vi "BuildPlotsOneGraph.vi"(0 "PlotCommand":string, 1 "Desired Legends":string[](array[string]), 2 "Error Bar Type":T1=enum."Standard Error", 5 "Plotstyles":T3[](array[typedef]) {"LineType" min=1 max=6 step=1; "LineWidth" min=1 max=6 step=1; "PointSize" min=0 step=0.1}, 7 "PlotNamesNeed $$?":bool=TRUE, 9 "Plot Legends":string[](array[string]), 11 "PlotArray":cluster{dbl[], dbl[]}[](array[cluster]), 12 "Legend":string[](array[string]), 13 "Error Bar Cluster":T2[](array[typedef])) -> (4 "String out":string, 6 "Xspan":cluster{"Max":dbl, "Min":dbl}, 10 "Yspan":cluster{"Max":dbl, "Min":dbl})   [LabVIEW 2018]
uses:
  plotstyle.ctl
  Error_bars.ctl
  Error bar Type.ctl
  Results_plotter_Global.vi
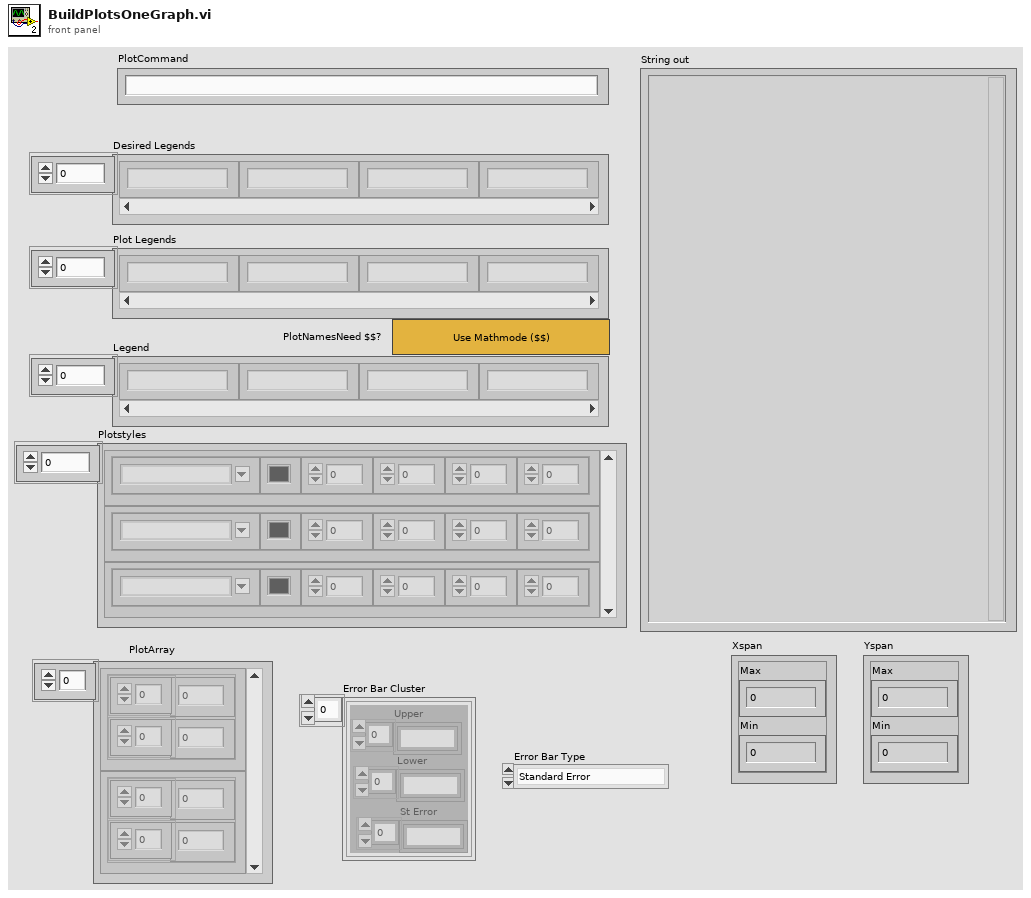
[diagram p1: front panel]
types:
  T1 = typedef "Error bar Type.ctl" = enum16{"None", "Standard Error", "Separate upper and lower"}
  T2 = typedef "Error_bars.ctl" = cluster{"Upper":string[], "Lower":string[], "St Error":string[]}
  T3 = typedef "plotstyle.ctl" = cluster{"Style":string, "Color":u32, "PointType":i32, "PointSize":sgl, "LineWidth":sgl, "LineType":u8}
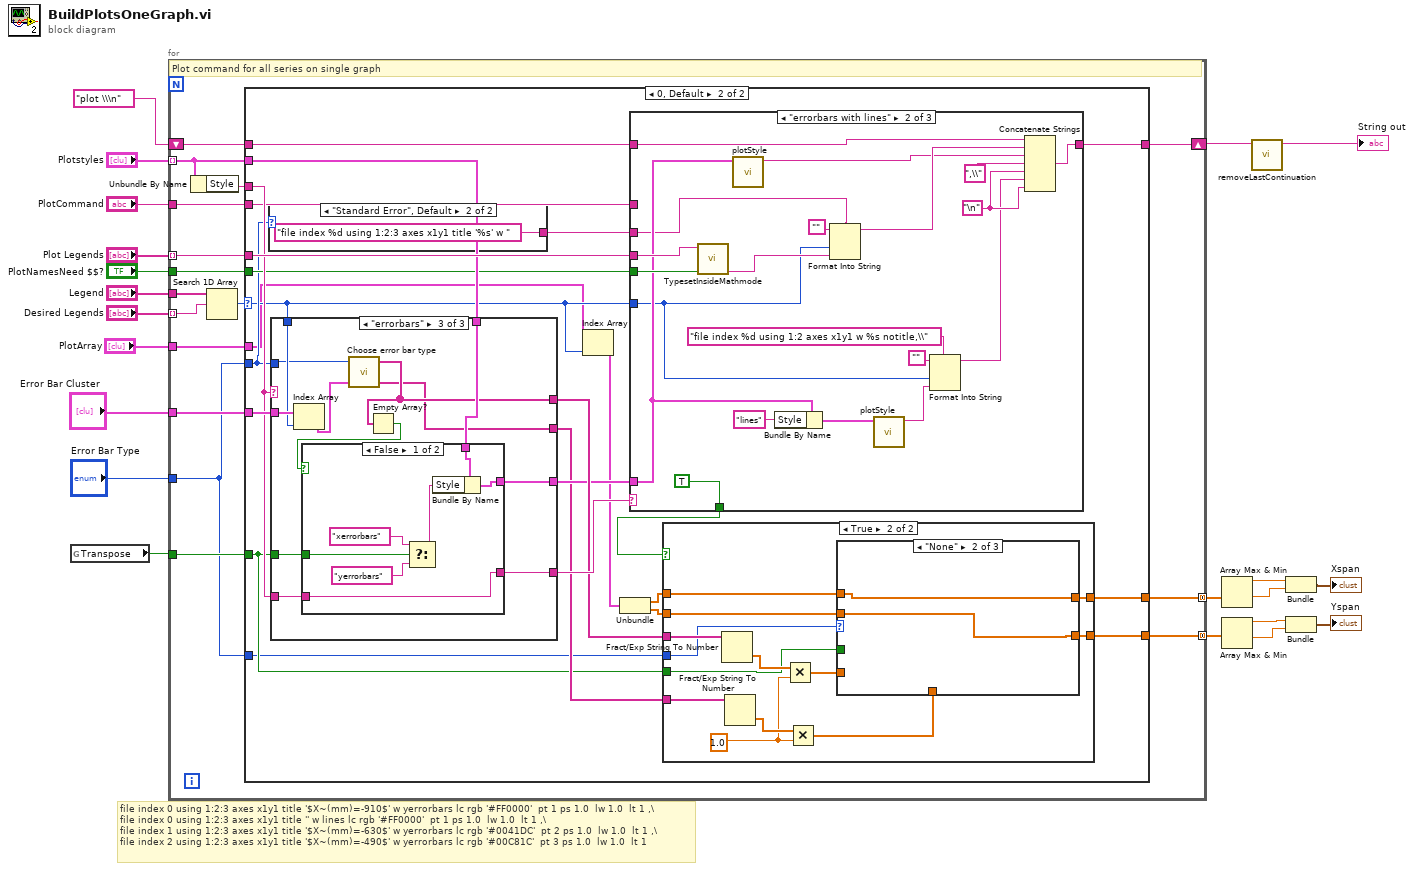
[diagram p0: block diagram]
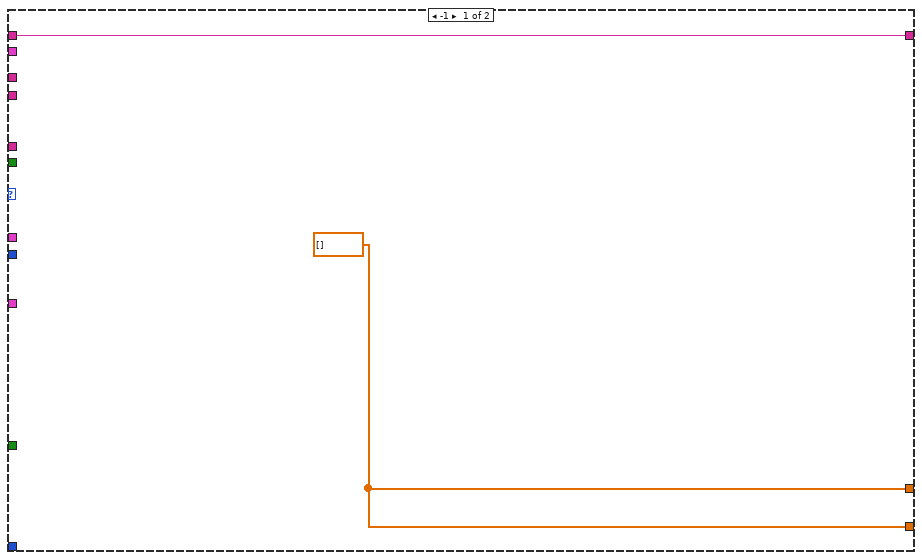
[diagram p2: hidden frame]
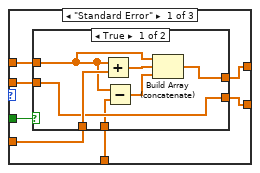
[diagram p4: hidden frame]
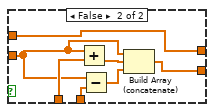
[diagram p5: hidden frame]
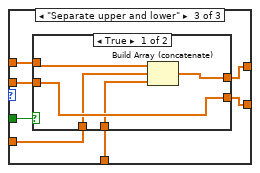
[diagram p6: hidden frame]
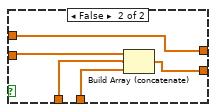
[diagram p7: hidden frame]
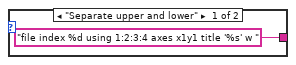
[diagram p8: hidden frame]
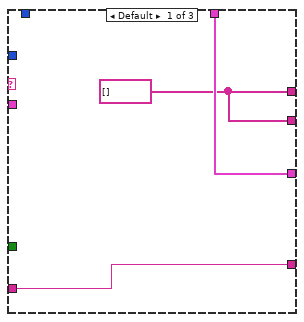
[diagram p9: hidden frame]
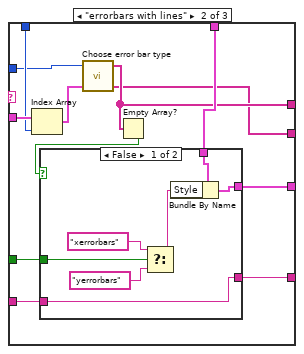
[diagram p10: hidden frame]
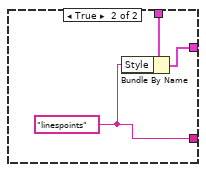
[diagram p11: hidden frame]
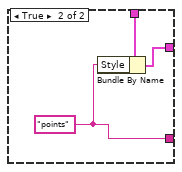
[diagram p12: hidden frame]
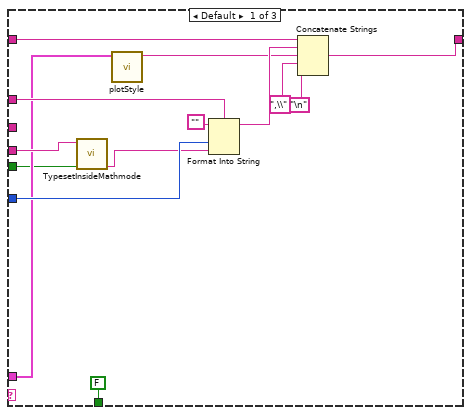
[diagram p13: hidden frame]
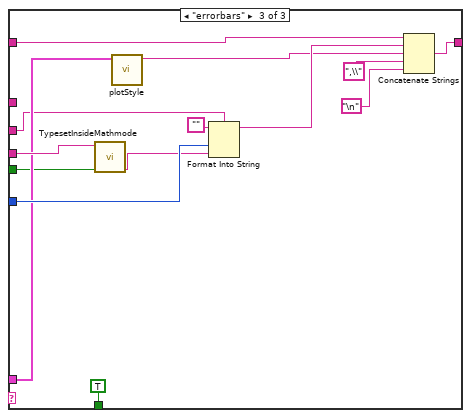
[diagram p14: hidden frame]
diagram:
  # "file index 0 using 1:2:3 axes x1y1 title '$X~(mm)=-910$' w yerrorbars lc rgb '#FF0000'  pt 1 ps 1.0  lw 1.0  lt 1 ,\\\nfile index 0 using 1:2:3 axes x1y1 title '' w lines lc rgb '#FF0000'  pt 1 ps 1.0  lw 1.0  lt 1 ,\\\nfile index 1 using 1:2:3 axes x1y1 title '$X~(mm)=-630$' w yerrorbars lc rgb '#0041DC'  pt 2 ps 1.0  lw 1.0  lt 1 ,\\\nfile index 2 using 1:2:3 axes x1y1 title '$X~(mm)=-490$' w yerrorbars lc rgb '#00C81C'  pt 3 ps 1.0  lw 1.0  lt 1"
  n1 = global read "Results_plotter_Global.vi" "Transpose"() -> (w3:bool)
  n2 = for {
    tunnel: "Plotstyles" -> [w27] mode=indexing
    tunnel: "Plot Legends" -> [w35] mode=indexing
    shift-right: [w36] -> w19
    shift-left: "plot \\\n" -> [w37]
    tunnel: "Desired Legends" -> [w33] mode=indexing
    tunnel: "Legend" -> [w34]
    tunnel: "PlotCommand" -> [w31]
    tunnel: "PlotArray" -> [w30]
    tunnel: [w29] -> w12 mode=concatenating
    tunnel: [w28] -> w11 mode=concatenating
    tunnel: "Error Bar Cluster" -> [w25]
    tunnel: w3 -> [w24]
    tunnel: "PlotNamesNeed $$?" -> [w23]
    tunnel: "Error Bar Type" -> [w22]
    # "Plot command for all series on single graph"
    n3 = Unbundle By Name(w27) -> ("Style"=w26:string)
    n4 = Search 1D Array(1D array=w34, element=w33) -> (index of element=w32:i32)  [unwired: 1 in]
    n5 = case shown="0, Default" w32 {
      selector: w32 -> [_ w46]
      tunnel: w27 -> [_ w59]
      tunnel: w37 -> [w39 w63]
      tunnel: [w39 w62] -> w36
      tunnel: w35 -> [_ w61]
      tunnel: w31 -> [_ w56]
      tunnel: w30 -> [_ w45]
      tunnel: [w38 w41] -> w29
      tunnel: [w38 w40] -> w28
      tunnel: w26 -> [_ w57]
      tunnel: w25 -> [_ w60]
      tunnel: w24 -> [_ w48]
      tunnel: w23 -> [_ w55]
      tunnel: w22 -> [_ w54]
      tunnel: w22 -> [_ w47]
      frame -1 {
        w38 = dbl[] []
      }
      frame 0, Default {
        n6 = case shown="\"Standard Error\", Default" w54 {
          tunnel: ["file index %d using 1:2:3:4 axes x1y1 title '%s' w " ("format string") "file index %d using 1:2:3 axes x1y1 title '%s' w " ("format string")] -> w53
          frame "Separate upper and lower" {
          }
          frame "Standard Error", Default {
          }
        }
        n7 = case shown="\"errorbars\"" w57 {
          tunnel: w60 -> [_ w135 w157]
          tunnel: w59 -> [w123 w131 w153]
          tunnel: [w123 w130 w152] -> w50
          tunnel: [w122 w133 w155] -> w58
          tunnel: w48 -> [_ w132 w154]
          tunnel: w57 -> [w122 w129 w151]
          tunnel: w46 -> [_ w128 w150]
          tunnel: [w121 w125 w147] -> w51
          tunnel: w54 -> [_ w126 w148]
          tunnel: [w121 w124 w146] -> w49
          frame Default {
            w121 = string[] []
          }
          frame "errorbars with lines" {
            n8 = Index Array(array=w135, index=w128) -> (element=w127:T2)
            n9 = call "Choose error bar type.vi"("Error_bars"=w127, "Error Bar Type"=w126) -> ("Lower"=w124:string[], "Upper"=w125:string[])  [unwired: 1 in, 1 out]
            n10 = Empty Array?(array=w125) -> (empty?=w134:bool)
            n11 = case shown="False" w134 {
              tunnel: [w136 w143] -> w133
              tunnel: w132 -> [w140 _]
              tunnel: w131 -> [w139 w145]
              tunnel: [w138 w144] -> w130
              tunnel: w129 -> [w136 _]
              frame False {
                n12 = Select(t="xerrorbars", s=w140, f="yerrorbars") -> (s? t:f=w137:string)
                n13 = Bundle By Name(cluster=w139, "Style"=w137) -> (w138:T3)
              }
              frame True {
                w143 = "linespoints" ("Style")
                n14 = Bundle By Name(cluster=w145, "Style"=w143) -> (w144:T3)
              }
            }
          }
          frame "errorbars" {
            n15 = Index Array(array=w157, index=w150) -> (element=w149:T2)
            n16 = call "Choose error bar type.vi"("Error_bars"=w149, "Error Bar Type"=w148) -> ("Lower"=w146:string[], "Upper"=w147:string[])  [unwired: 1 in, 1 out]
            n17 = Empty Array?(array=w147) -> (empty?=w156:bool)
            n18 = case shown="False" w156 {
              tunnel: [w158 w165] -> w155
              tunnel: w154 -> [w162 _]
              tunnel: w153 -> [w161 w167]
              tunnel: [w160 w166] -> w152
              tunnel: w151 -> [w158 _]
              frame False {
                n19 = Select(t="xerrorbars", s=w162, f="yerrorbars") -> (s? t:f=w159:string)
                n20 = Bundle By Name(cluster=w161, "Style"=w159) -> (w160:T3)
              }
              frame True {
                w165 = "points" ("Style")
                n21 = Bundle By Name(cluster=w167, "Style"=w165) -> (w166:T3)
              }
            }
          }
        }
        n22 = Index Array(array=w45, index=w46) -> (element=w44:cluster{dbl[], dbl[]})
        n23 = Unbundle(w44) -> (w43:dbl[], w42:dbl[])
        n24 = case shown="\"errorbars with lines\"" w58 {
          tunnel: w63 -> [w176 w197 w211]
          tunnel: [w171 w196 w210] -> w62
          tunnel: w56 -> [w175 _ _]
          tunnel: w46 -> [w174 w183 w208]
          tunnel: w61 -> [w173 w195 w209]
          tunnel: w50 -> [w172 w185 w206]
          tunnel: w55 -> [w170 w187 w205]
          tunnel: w53 -> [_ w184 w203]
          tunnel: [FALSE TRUE TRUE] -> w52
          frame Default {
            n25 = call "TypesetInsideMathmode.vi"("Needs $$?"=w170, "DirtyString"=w173) -> ("ChosenStringtype"=w169:string)  [unwired: 7 in, 2 out]
            n26 = call "plotStyle.vi"("plotSpec"=w172) -> ("String"=w178:string)  [unwired: 10 in]
            n27 = Format Into String(format string=w175, initial string="", w174, w169) -> (resulting string=w179:string)  [unwired: 1 in, 1 out]
            n28 = Concatenate Strings(w176, w179, w178, ",\\" ("string"), "\n") -> (w171:string)
          }
          frame "errorbars with lines" {
            w189 = "\n"
            n29 = call "TypesetInsideMathmode.vi"("Needs $$?"=w187, "DirtyString"=w195) -> ("ChosenStringtype"=w186:string)  [unwired: 7 in, 2 out]
            n30 = call "plotStyle.vi"("plotSpec"=w185) -> ("String"=w198:string)  [unwired: 10 in]
            n31 = Bundle By Name(cluster=w185, "Style"="lines") -> (w192:T3)
            n32 = Format Into String(format string=w184, initial string="", w183, w186) -> (resulting string=w199:string)  [unwired: 1 in, 1 out]
            n33 = call "plotStyle.vi"("plotSpec"=w192) -> ("String"=w190:string)  [unwired: 10 in]
            n34 = Format Into String(format string="file index %d using 1:2 axes x1y1 w %s notitle,\\", initial string="", w183, w190) -> (resulting string=w188:string)  [unwired: 1 in, 1 out]
            n35 = Concatenate Strings(w197, w199, w198, ",\\" ("string"), w189, w188, w189) -> (w196:string)
          }
          frame "errorbars" {
            n36 = call "TypesetInsideMathmode.vi"("Needs $$?"=w205, "DirtyString"=w209) -> ("ChosenStringtype"=w204:string)  [unwired: 7 in, 2 out]
            n37 = call "plotStyle.vi"("plotSpec"=w206) -> ("String"=w212:string)  [unwired: 10 in]
            n38 = Format Into String(format string=w203, initial string="", w208, w204) -> (resulting string=w213:string)  [unwired: 1 in, 1 out]
            n39 = Concatenate Strings(w211, w213, w212, ",\\" ("string"), "\n") -> (w210:string)
          }
        }
        n40 = case shown="True" w52 {
          tunnel: w51 -> [_ w74]
          tunnel: w49 -> [_ w73]
          tunnel: w48 -> [_ w71]
          tunnel: w47 -> [_ w70]
          tunnel: w43 -> [w65 w69]
          tunnel: w42 -> [w64 w68]
          tunnel: [w65 w67] -> w41
          tunnel: [w64 w66] -> w40
          frame False {
          }
          frame True {
            w72 = 1.0
            n41 = Fract/Exp String To Number(string=w74) -> (number=w78:dbl[])  [unwired: 3 in, 1 out]
            n42 = Fract/Exp String To Number(string=w73) -> (number=w76:dbl[])  [unwired: 3 in, 1 out]
            n43 = Multiply(x=w78, y=w72) -> (x*y=w77:dbl[])
            n44 = Multiply(x=w76, y=w72) -> (x*y=w75:dbl[])
            n45 = case shown="\"None\"" w70 {
              tunnel: w69 -> [w85 w101 w108]
              tunnel: w77 -> [w84 _ w107]
              tunnel: w68 -> [w83 w100 w106]
              tunnel: w75 -> [w82 _ w105]
              tunnel: w71 -> [w81 _ w104]
              tunnel: [w80 w101 w103] -> w67
              tunnel: [w79 w100 w102] -> w66
              frame "Standard Error" {
                n46 = case shown="True" w81 {
                  tunnel: w85 -> [w86 w96]
                  tunnel: w84 -> [w90 w97]
                  tunnel: [w89 w96] -> w80
                  tunnel: [w88 w95] -> w79
                  tunnel: w83 -> [w88 w93]
                  tunnel: w82 -> [w87 w94]
                  frame True {
                    n47 = Add(x=w86, y=w90) -> (x+y=w91:dbl[])
                    n48 = Subtract(x=w86, y=w87) -> (x-y=w92:dbl[])
                    n49 = Build Array (concatenate)(w86, w91, w92) -> (w89:dbl[])
                  }
                  frame False {
                    n50 = Add(x=w93, y=w97) -> (x+y=w98:dbl[])
                    n51 = Subtract(x=w93, y=w94) -> (x-y=w99:dbl[])
                    n52 = Build Array (concatenate)(w93, w98, w99) -> (w95:dbl[])
                  }
                }
              }
              frame "None" {
              }
              frame "Separate upper and lower" {
                n53 = case shown="True" w104 {
                  tunnel: w108 -> [w109 w118]
                  tunnel: w107 -> [w111 w116]
                  tunnel: [w113 w118] -> w103
                  tunnel: [w112 w117] -> w102
                  tunnel: w106 -> [w112 w114]
                  tunnel: w105 -> [w110 w115]
                  frame True {
                    n54 = Build Array (concatenate)(w109, w111, w110) -> (w113:dbl[])
                  }
                  frame False {
                    n55 = Build Array (concatenate)(w114, w116, w115) -> (w117:dbl[])
                  }
                }
              }
            }
          }
        }
      }
    }
  }
  n56 = Array Max & Min(array=w12) -> (max value=w9:dbl, min value=w8:dbl)  [unwired: 2 out]
  n57 = Array Max & Min(array=w11) -> (max value=w7:dbl, min value=w6:dbl)  [unwired: 2 out]
  n58 = call "removeLastContinuation.vi"("String in"=w19) -> ("String out"=→"String out":string)  [unwired: 10 in]
  n59 = Bundle(w9, w8) -> (→"Xspan":cluster{dbl, dbl})  [unwired: 1 in]
  n60 = Bundle(w7, w6) -> (→"Yspan":cluster{dbl, dbl})  [unwired: 1 in]
